vi "Set_Logging_All.vi"() -> ()   [LabVIEW 2016, in "data.citadel.lvclass"]
uses:
  data.citadel.lvclass
  <vilib>/lvdsc/NI_DSC.lvlib
panel:
  in  "IP or PC Name":string="HousesOfTheHoly"
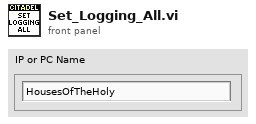
[diagram p1: front panel]
types:
  T1 = cluster{"enable? (F)":bool, "data type (deprecated)":enum32{"U32 Bit Field", "Boolean", "Double", "String"}, "log data? (F)":bool, "log alarms & events? (F)":bool, "value resolution (for Float variables only)":dbl, "value deadband (for Float variables only)":dbl, "string logging format (for String variables only)":u32}
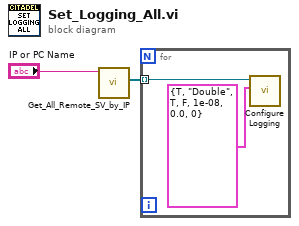
[diagram p0: block diagram]
diagram:
  n1 = call "Get_All_Remote_SV_by_IP.vi"("IP Address"="IP or PC Name") -> ("Shared Variable List"=w1:refnum<k21>[])  [unwired: 8 in, 2 out]
  n2 = for {
    tunnel: w1 -> [w3] mode=indexing
    n3 = call <vilib>:"Configure Logging.vi"("logging settings"=T1 {"enable? (F)"=TRUE, "data type (deprecated)"=enum."Double", "log data? (F)"=TRUE, "log alarms & events? (F)"=FALSE, "value resolution (for Float variables only)"=1e-08, "value deadband (for Float variables only)"=0.0, "string logging format (for String variables only)"=0}, "variable reference in"=w3) -> ()  [unwired: 8 in, 2 out]
  }
